vi "simulation.vi"() -> ()   [LabVIEW 2021]
doc: "This is the TCP server VI that supports multiple connections from client VIs."
panel:
  in  "Pinky Finger":dbl(knob) scale=0.0..90.0
  in  "Ring Finger":dbl(knob) scale=0.0..90.0
  in  "Middle Finger":dbl(knob) scale=0.0..90.0
  in  "Index Finger":dbl(knob) scale=0.0..90.0
  in  "Thumb":dbl(knob) scale=0.0..90.0
  out "Simulation Connected":bool
  out "Pinky Finger":dbl
  out "Ring Finger":dbl
  out "Middle Finger":dbl
  out "Index Finger":dbl
  in  "Stop":bool
  out "Thumb":dbl
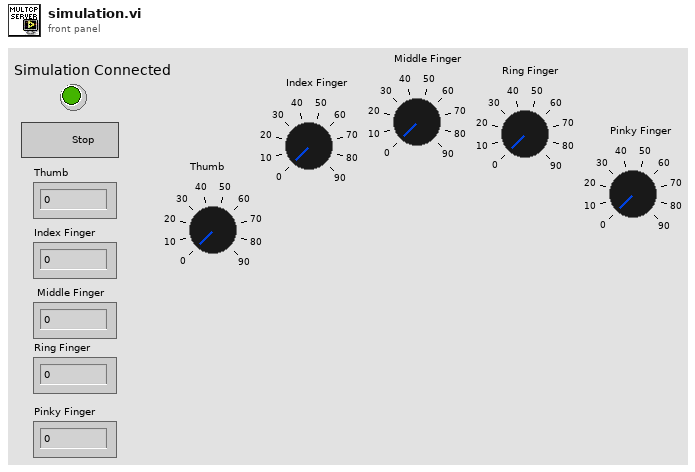
[diagram p1: front panel]
types:
  T1 = cluster{"Clients":refnum<k5>[], "Listener":refnum<k5>}
  T2 = enum16{"Initialize", "Status Check", "Send Data", "Stop"}
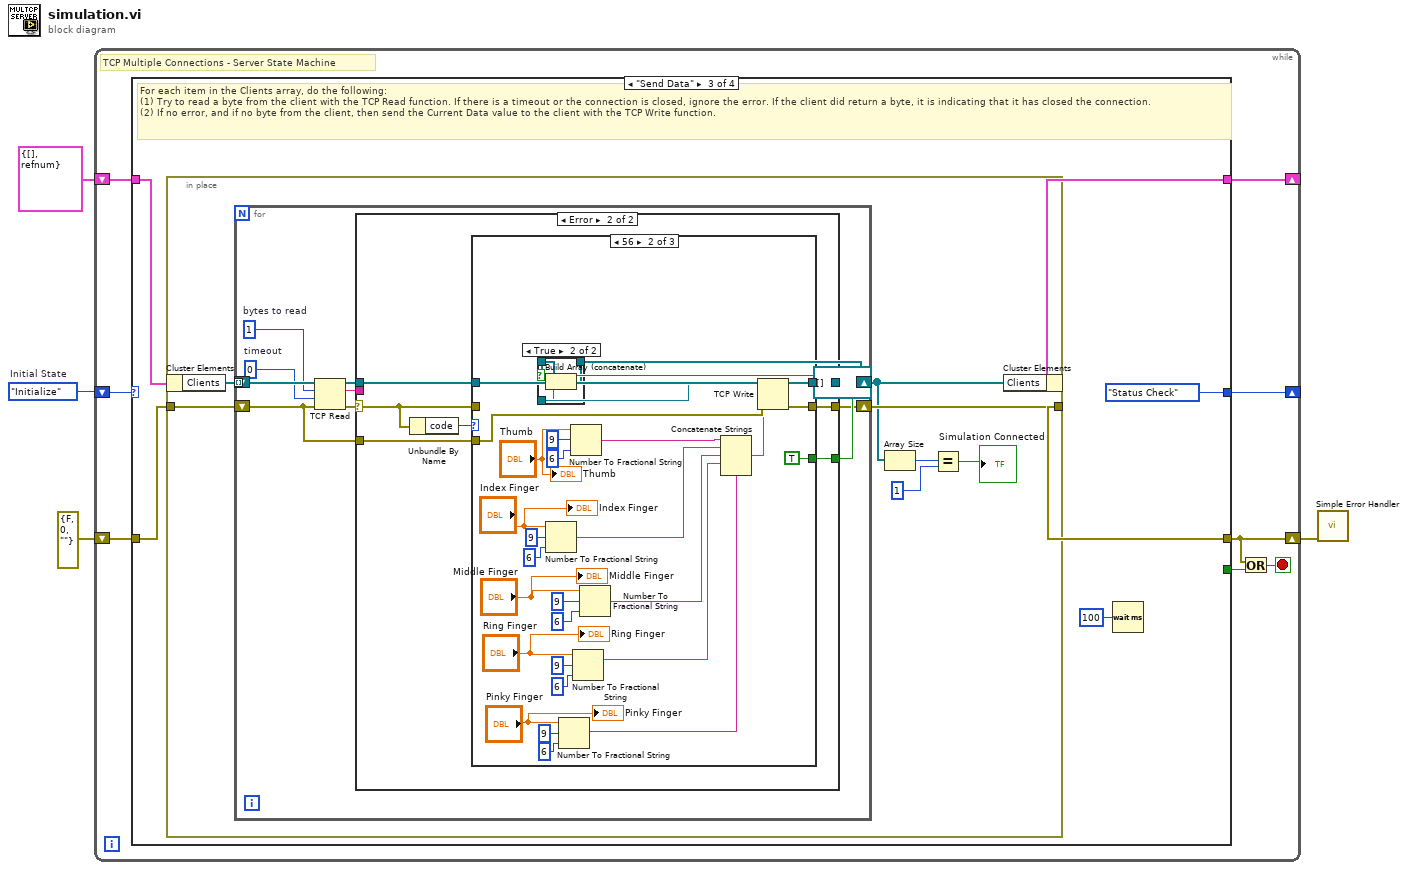
[diagram p0: block diagram]
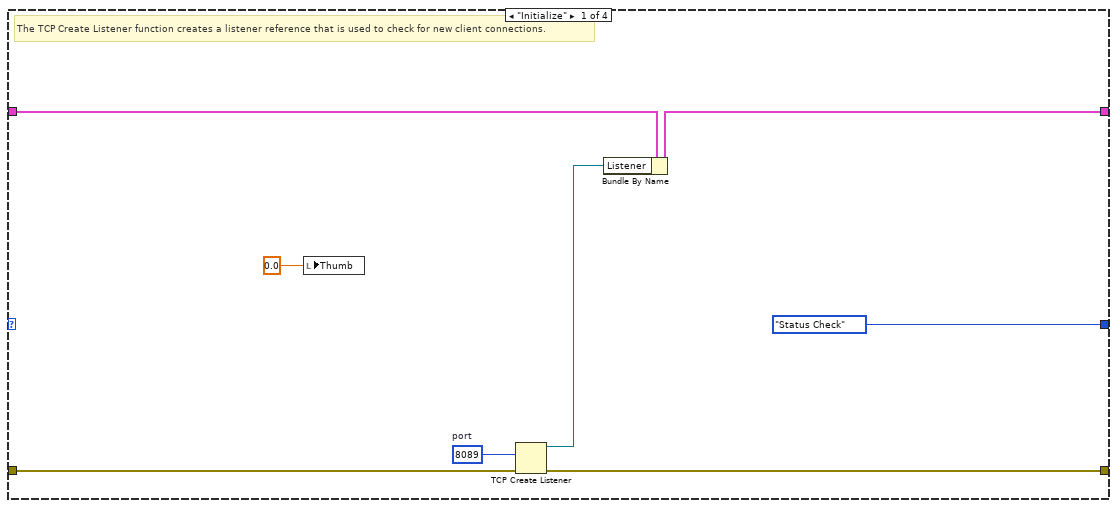
[diagram p2: hidden frame]
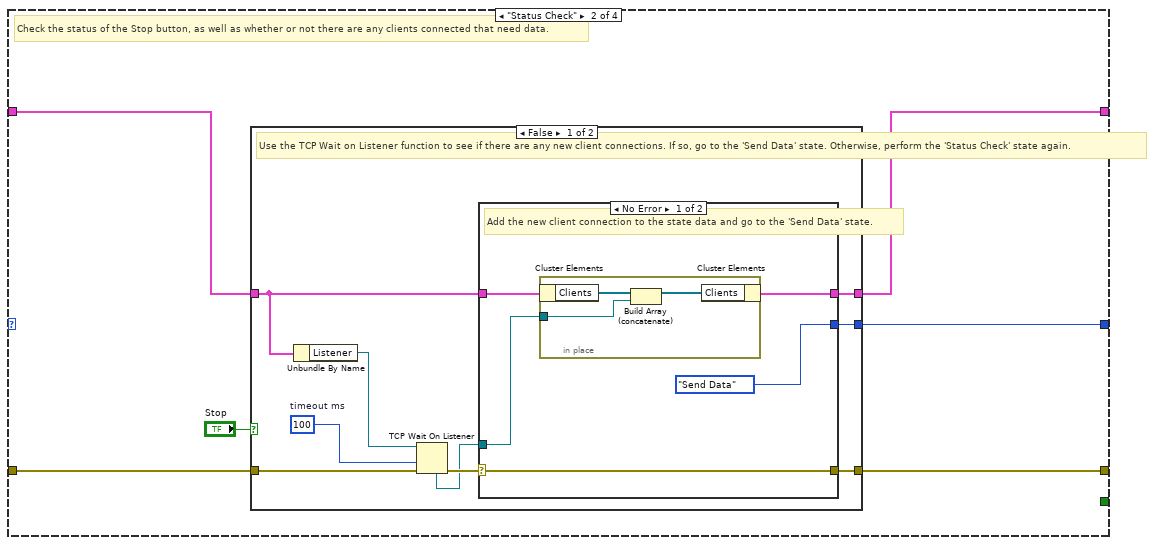
[diagram p3: hidden frame]
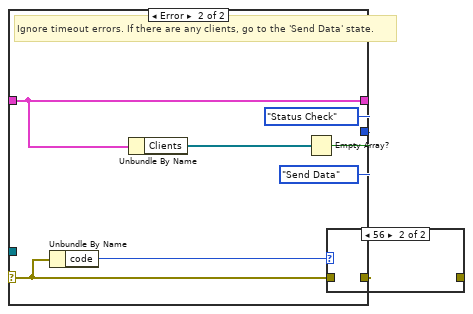
[diagram p4: hidden frame]
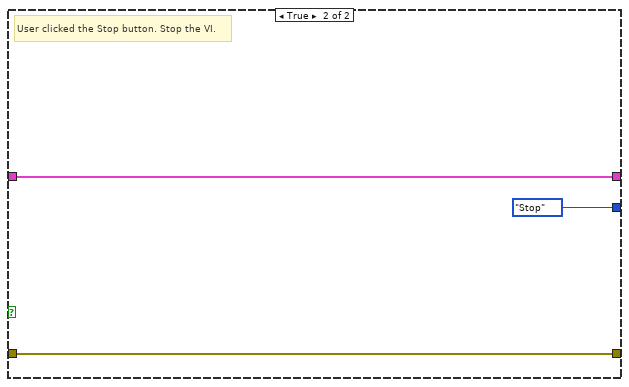
[diagram p6: hidden frame]
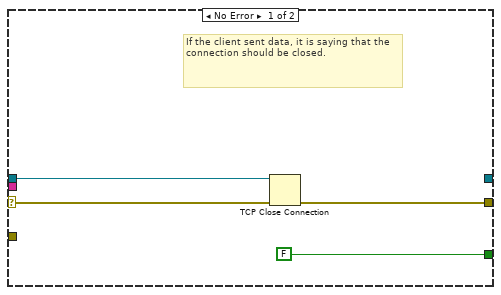
[diagram p8: hidden frame]
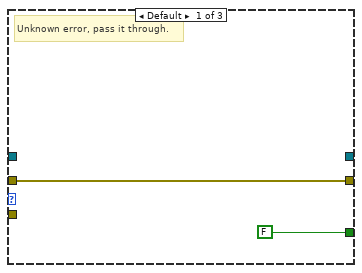
[diagram p9: hidden frame]
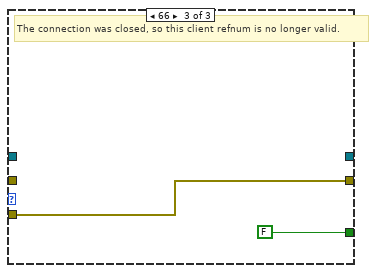
[diagram p10: hidden frame]
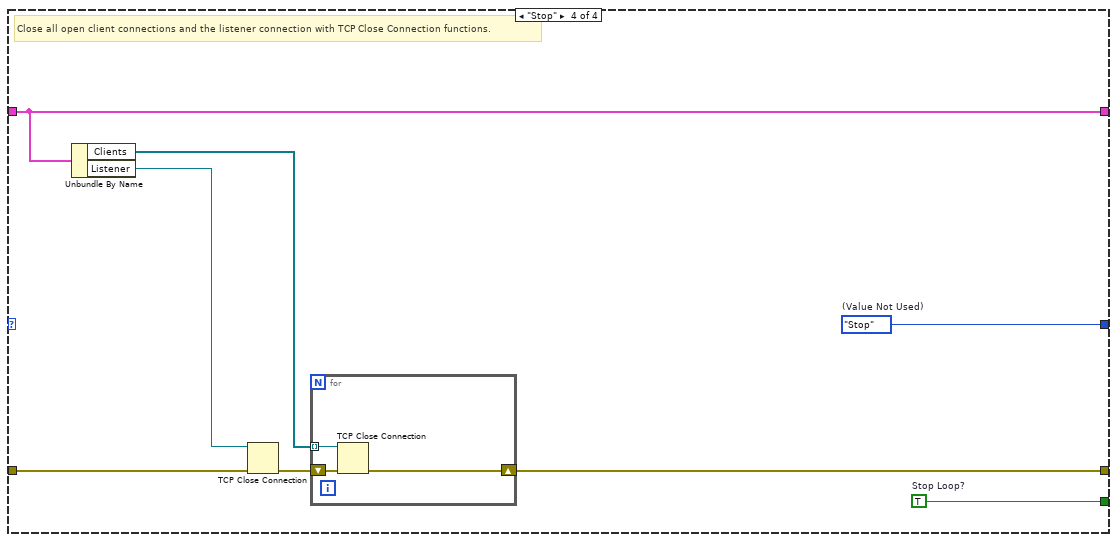
[diagram p11: hidden frame]
diagram:
  w4 = T2."Initialize"  # Initial State
  n1 = while {
    shift-right: [w11] -> _
    shift-left: w4 -> [w12]
    shift-right: [w9] -> _
    shift-left: T1 {"Clients"=[], "Listener"=refnum} ("Data") -> [w10]
    shift-right: [w5] -> w1
    shift-left: errorcluster {"status"=FALSE, "code"=0, "source"=""} ("error constant") -> [w8]
    stop <- w6 stop-if-true
    # "TCP Multiple Connections - Server State Machine"
    n2 = case shown="\"Send Data\"" w12 {
      tunnel: [T2."Status Check" ("States") w26 T2."Status Check" ("States") w129] -> w11
      tunnel: [_ _ _ w136] -> w7
      tunnel: w10 -> [w18 w22 w61 w135]
      tunnel: [w17 w21 w60 w135] -> w9
      tunnel: w8 -> [w20 w25 w63 w134]
      tunnel: [w19 w24 w62 w132] -> w5
      frame "Initialize" {
        w15 = u16 8089  # port
        # "The TCP Create Listener function creates a listener reference that is used to check for new client connections."
        n3 = local write "Thumb"(0.0 ("Current Data")) -> ()
        n4 = TCP Create Listener(8:w20, 10:w15) -> (0:w19:errorcluster, 3:w16:refnum<k5>)  [unwired: 4 out]
        n5 = Bundle By Name(cluster=w18, "Listener"=w16) -> (w17:T1)
      }
      frame "Status Check" {
        # "Check the status of the Stop button, as well as whether or not there are any clients connected that need data."
        n6 = case shown="False" "Stop" {
          tunnel: [w35 T2."Stop" ("States")] -> w26
          tunnel: w25 -> [w34 w57]
          tunnel: [w27 w57] -> w24
          tunnel: w22 -> [w30 w56]
          tunnel: [w29 w56] -> w21
          frame False {
            w33 = 100  # timeout ms
            # "Use the TCP Wait on Listener function to see if there are any new client connections. If so, go to the 'Send Data' state. Otherwise, perform the 'Status Check' state again."
            n7 = Unbundle By Name(w30) -> ("Listener"=w28:refnum<k5>)
            n8 = TCP Wait On Listener(8:w34, 9:w33, 11:w28) -> (0:w32:errorcluster, 4:w31:refnum<k5>)  [unwired: 4 out]
            n9 = case shown="No Error" w32 {
              selector: w32 -> [w38 w52]
              tunnel: [T2."Send Data" ("States") w46] -> w35
              tunnel: w31 -> [w39 _]
              tunnel: w30 -> [w40 w49]
              tunnel: [w37 w49] -> w29
              tunnel: [w38 w50] -> w27
              frame No Error {
                # "Add the new client connection to the state data and go to the 'Send Data' state."
                n10 = in-place {
                  in-place-border: w39 -> [w41]
                  n11 = in-place-cluster #1(w40) -> ("Clients"=w43:refnum<k5>[])
                  n12 = Build Array (concatenate)(w43, w41) -> (w42:refnum<k5>[])
                  n13 = in-place-cluster #1("Clients"=w42) -> (w37:T1)
                }
              }
              frame Error {
                # "Ignore timeout errors. If there are any clients, go to the 'Send Data' state."
                n14 = Unbundle By Name(w52) -> ("code"=w51:i32)
                n15 = Unbundle By Name(w49) -> ("Clients"=w48:refnum<k5>[])
                n16 = Empty Array?(array=w48) -> (empty?=w47:bool)
                n17 = case shown="56" w51 {
                  tunnel: w52 -> [w53 _]
                  tunnel: [w53 w54] -> w50
                  frame Default {
                  }
                  frame 56 {
                    w54 = errorcluster {"status"=FALSE, "code"=0, "source"=""}  # no error
                  }
                }
                n18 = Select(t=T2."Status Check" ("States"), s=w47, f=T2."Send Data" ("States")) -> (s? t:f=w46:T2)
              }
            }
          }
          frame True {
            # "User clicked the Stop button. Stop the VI."
          }
        }
      }
      frame "Send Data" {
        # "For each item in the Clients array, do the following:\n(1) Try to read a byte from the client with the TCP Read function. If there is a timeout or the connection is closed, ignore the error. If the client did return a byte, it is indicating that it has closed the connection.\n(2) If no error, and if no byte from the client, then send the Current Data value to the client with the TCP Write function."
        n19 = in-place {
          in-place-border: w63 -> [w71]
          in-place-border: [w70] -> w62
          n20 = in-place-cluster #2(w61) -> ("Clients"=w69:refnum<k5>[])
          n21 = for {
            tunnel: w69 -> [w83] mode=indexing
            shift-right: [w75] -> w70
            shift-left: w71 -> [w74]
            shift-right: [w72] -> w68
            shift-left: refnum<k5>[] [] ("Array") -> [w73]
            w80 = 0  # timeout
            w81 = 1  # bytes to read
            n22 = TCP Read(connection ID=w83, bytes to read=w81, error in (no error)=w74, 9:w80) -> (connection ID out=w82:refnum<k5>, data out=w78:string, error out=w79:errorcluster)  [unwired: 1 out]
            n23 = case shown="Error" w79 {
              selector: w79 -> [w90 w97]
              tunnel: w82 -> [w91 w94]
              tunnel: w78 -> [_ _]
              tunnel: [_ w92] -> w77
              tunnel: [FALSE w93] -> w76
              tunnel: [w88 w96] -> w75
              tunnel: w74 -> [_ w95]
              frame No Error {
                # "If the client sent data, it is saying that the connection should be closed."
                # "If the client sent data, it is saying that the connection should be closed."
                n24 = TCP Close Connection(connection ID=w91, error in (no error)=w90) -> (error out=w88:errorcluster)  [unwired: 2 out]
              }
              frame Error {
                # "Ignore connection closed and timeout errors"
                n25 = Unbundle By Name(w97) -> ("code"=w98:i32)
                n26 = case shown="56" w98 {
                  tunnel: w97 -> [w100 _ _]
                  tunnel: [w100 w126 w128] -> w96
                  tunnel: w95 -> [_ w122 w128]
                  tunnel: w94 -> [_ w125 _]
                  tunnel: [FALSE TRUE FALSE] -> w93
                  tunnel: [_ w124 _] -> w92
                  frame Default {
                    # "Unknown error, pass it through."
                  }
                  frame 56 {
                    n27 = Number To Fractional String(number="Index Finger", width (-)=i16 9, precision (6)=i16 6) -> (F-format string=w119:string)  [unwired: 1 in]
                    n28 = Number To Fractional String(number="Pinky Finger", width (-)=i16 9, precision (6)=i16 6) -> (F-format string=w116:string)  [unwired: 1 in]
                    n29 = Number To Fractional String(number="Thumb", width (-)=i16 9, precision (6)=i16 6) -> (F-format string=w120:string)  [unwired: 1 in]
                    n30 = Number To Fractional String(number="Ring Finger", width (-)=i16 9, precision (6)=i16 6) -> (F-format string=w117:string)  [unwired: 1 in]
                    n31 = Number To Fractional String(number="Middle Finger", width (-)=i16 9, precision (6)=i16 6) -> (F-format string=w118:string)  [unwired: 1 in]
                    n32 = Concatenate Strings(w120, w119, w118, w117, w116) -> (w121:string)
                    n33 = TCP Write(connection ID=w125, data in=w121, error in (no error)=w122) -> (connection ID out=w124:refnum<k5>, error out=w126:errorcluster)  [unwired: 2 out]
                    "Thumb" <- "Thumb"
                    "Index Finger" <- "Index Finger"
                    "Middle Finger" <- "Middle Finger"
                    "Ring Finger" <- "Ring Finger"
                    "Pinky Finger" <- "Pinky Finger"
                  }
                  frame 66 {
                    # "The connection was closed, so this client refnum is no longer valid."
                  }
                }
              }
            }
            n34 = case shown="True" w76 {
              tunnel: w73 -> [w84 w86]
              tunnel: w77 -> [_ w85]
              tunnel: [w84 w87] -> w72
              frame False {
              }
              frame True {
                n35 = Build Array (concatenate)(w86, w85) -> (w87:refnum<k5>[])
              }
            }
          }
          n36 = Array Size(array=w68) -> (size(s)=w66:i32)
          n37 = Equal?(x=w66, y=1) -> (x = y?=→"Simulation Connected":bool)
          n38 = in-place-cluster #2("Clients"=w68) -> (w60:T1)
        }
        n39 = Wait (ms)(milliseconds to wait=u32 100) -> ()  [unwired: 1 out]
      }
      frame "Stop" {
        w129 = T2."Stop"  # (Value Not Used)
        w136 = TRUE  # Stop Loop?
        # "Close all open client connections and the listener connection with TCP Close Connection functions."
        n40 = Unbundle By Name(w135) -> ("Clients"=w133:refnum<k5>[], "Listener"=w130:refnum<k5>)
        n41 = TCP Close Connection(connection ID=w130, error in (no error)=w134) -> (error out=w131:errorcluster)  [unwired: 1 in, 1 out]
        n42 = for {
          shift-right: [w138] -> w132
          shift-left: w131 -> [w139]
          tunnel: w133 -> [w137] mode=indexing
          n43 = TCP Close Connection(connection ID=w137, error in (no error)=w139) -> (error out=w138:errorcluster)  [unwired: 1 in, 1 out]
        }
      }
    }
    n44 = Or(x=w5, y=w7) -> (x .or. y?=w6:bool)
  }
  n45 = call <vilib>:"Simple Error Handler.vi"("error in (no error)"=w1) -> ()  [unwired: 4 in, 5 out]
